vi "-8300 Source with Invalid File Extension--error.vi"(8 "error in (no error)":errorcluster, 11 "Source":string) -> (0 "error out":errorcluster)   [LabVIEW 2024, in "Instrument Factory.lvclass"]
uses:
  Instrument Factory.lvclass
  Instrument Factory.lvclass/Instrument Factory.ctl
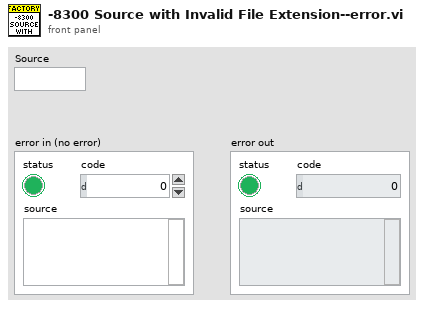
[diagram p1: front panel]
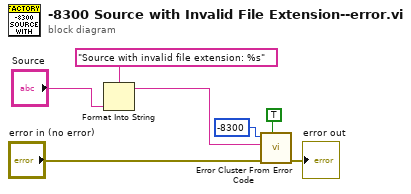
[diagram p0: block diagram]
diagram:
  n1 = Format Into String(format string="Source with invalid file extension: %s", "Source") -> (resulting string=w3:string)  [unwired: 2 in, 1 out]
  n2 = call <vilib>:"Error Cluster From Error Code.vi"("show call chain? (False)"=TRUE, "error in (no error)"="error in (no error)", "error message (\"\")"=w3, "error code (0)"=-8300) -> ("error out"=→"error out":errorcluster)  [unwired: 5 in]
